vi "Read Debug.vi"(11 "Ancestral Actor in":refnum<class "Ancestral Actor.lvclass">) -> (2 "Debug":bool, 3 "Ancestral Actor out":refnum<class "Ancestral Actor.lvclass">)   [LabVIEW 2016, in "Stream Actor.lvlib" / "Ancestral Actor.lvclass"]
uses:
  <userlib>/Composed Systems/Stream/Actor/Actor Class/Ancestral Actor.lvclass
  <userlib>/Composed Systems/Stream/Actor/Actor Class/Ancestral Actor.lvclass/Ancestral Actor.ctl
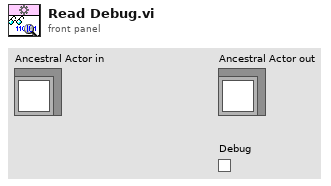
[diagram p1: front panel]
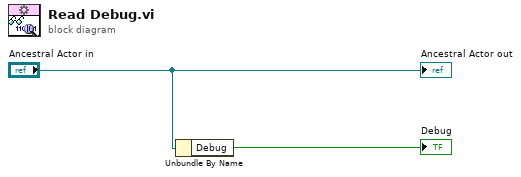
[diagram p0: block diagram]
diagram:
  n1 = Unbundle By Name("Ancestral Actor in") -> ("Debug"=→"Debug":bool)
  "Ancestral Actor out" <- "Ancestral Actor in"
